vi "get filter from UI inputs.vi"(9 "NOT":bool, 10 "Filter Value":string, 11 "Filter Type":T1) -> (3 "Filter out":refnum<class "Filter.lvclass">)   [LabVIEW 2016, in "RM.Server.lvlib"]
uses:
  RM.Server.lvlib
  Client/Test CD/FPGA RM Test Client/Source/System Explorer/Filters/Filter Parent/Filter.lvclass
  viz_filter.ctl
  Client/Test CD/FPGA RM Test Client/Source/System Explorer/Filters/RIO Device Filter/RIO Device Filter.lvclass
  Client/Test CD/FPGA RM Test Client/Source/System Explorer/Filters/Resource Name Filter/Resource Name Filter.lvclass
  Client/Test CD/FPGA RM Test Client/Source/System Explorer/Filters/Input Type Filter/Input Type Filter.lvclass
  Client/Test CD/FPGA RM Test Client/Source/System Explorer/Filters/NOT Filter/NOT Filter.lvclass
  Client/Test CD/FPGA RM Test Client/Source/System Explorer/Filters/Datatype Filter/Datatype Filter.lvclass
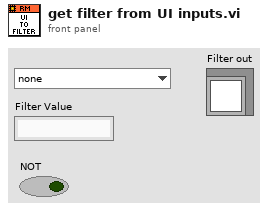
[diagram p1: front panel]
types:
  T1 = typedef "RM.Server.lvlib/viz_filter.ctl" = enum16{"none", "RIO Device", "Resource Name", "Input Type", "Datatype"}
  T2 = enum16{"Scalar Inputs", "Scalar Outputs", "Waveform Inputs", "Waveform Outputs"}
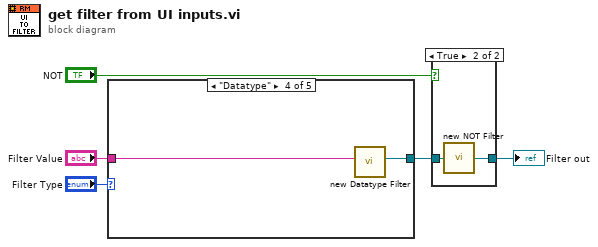
[diagram p0: block diagram]
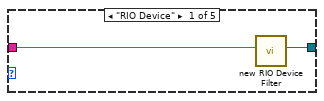
[diagram p3: hidden frame]
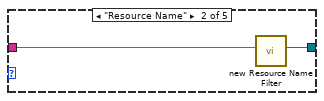
[diagram p4: hidden frame]
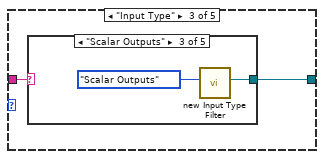
[diagram p5: hidden frame]
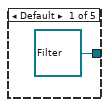
[diagram p6: hidden frame]
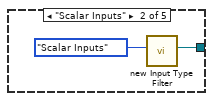
[diagram p7: hidden frame]
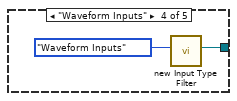
[diagram p8: hidden frame]
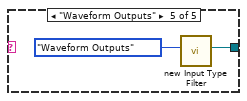
[diagram p9: hidden frame]
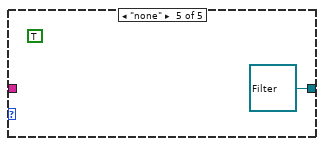
[diagram p10: hidden frame]
diagram:
  n1 = case shown="\"Datatype\"" "Filter Type" {
    tunnel: "Filter Value" -> [w7 w9 w11 w21 _]
    tunnel: [w6 w8 w10 w22 refnum<class "Filter.lvclass"> refnum ("Filter.lvclass")] -> w2
    frame "RIO Device" {
      n2 = call "new RIO Device Filter.vi"("RIO Device Name"=w7) -> ("RIO device filter out"=w6:refnum<class "Filter.lvclass">)  [unwired: 9 in]
    }
    frame "Resource Name" {
      n3 = call "new Resource Name Filter.vi"("Resource Name"=w9) -> ("resource name filter out"=w8:refnum<class "Filter.lvclass">)  [unwired: 10 in]
    }
    frame "Input Type" {
      n4 = case shown="\"Scalar Outputs\"" w11 {
        tunnel: [refnum<class "Filter.lvclass"> refnum ("datatype filter out") w14 w16 w18 w20] -> w10
        frame Default {
        }
        frame "Scalar Inputs" {
          n5 = call "new Input Type Filter.vi"("Input Type"=T2."Scalar Inputs" ("datatype")) -> ("input type filter out"=w14:refnum<class "Filter.lvclass">)  [unwired: 10 in]
        }
        frame "Scalar Outputs" {
          n6 = call "new Input Type Filter.vi"("Input Type"=T2."Scalar Outputs" ("datatype")) -> ("input type filter out"=w16:refnum<class "Filter.lvclass">)  [unwired: 10 in]
        }
        frame "Waveform Inputs" {
          n7 = call "new Input Type Filter.vi"("Input Type"=T2."Waveform Inputs" ("datatype")) -> ("input type filter out"=w18:refnum<class "Filter.lvclass">)  [unwired: 10 in]
        }
        frame "Waveform Outputs" {
          n8 = call "new Input Type Filter.vi"("Input Type"=T2."Waveform Outputs" ("datatype")) -> ("input type filter out"=w20:refnum<class "Filter.lvclass">)  [unwired: 10 in]
        }
      }
    }
    frame "Datatype" {
      n9 = call "new Datatype Filter.vi"("datatype"=w21) -> ("datatype filter out"=w22:refnum<class "Filter.lvclass">)  [unwired: 10 in]
    }
    frame "none" {
      (unwired) TRUE
    }
  }
  n10 = case shown="True" "NOT" {
    tunnel: w2 -> [w24 w26]
    tunnel: [w24 w25] -> w1
    frame False {
    }
    frame True {
      n11 = call "new NOT Filter.vi"("a"=w26) -> ("not a"=w25:refnum<class "Filter.lvclass">)  [unwired: 14 in]
    }
  }
  "Filter out" <- w1
